vi "Sel Biometry Average Standard Deviation.vi"(8 "error in (no error)":errorcluster caption="错误输入（无错误）", 9 "condition":string, 11 "connection reference":T2) -> (0 "error out":errorcluster caption="错误输出", 2 "Biometry_Average_Standard_Deviation":T1[](array[typedef]))   [LabVIEW 2015, in "Database Processing.lvlib"]
doc: "该模板用于创建子VI。"
uses:
  Database Processing.lvlib
  <vilib>/addons/database/Connection.llb/Conn ObjectReference.ctl
  Support/Table/Biometry Average Standard Deviation.ctl
  <vilib>/addons/database/_DB Variant To Data/Database Variant To Data.xnode
  <vilib>/addons/database/NI_Database_API.lvlib
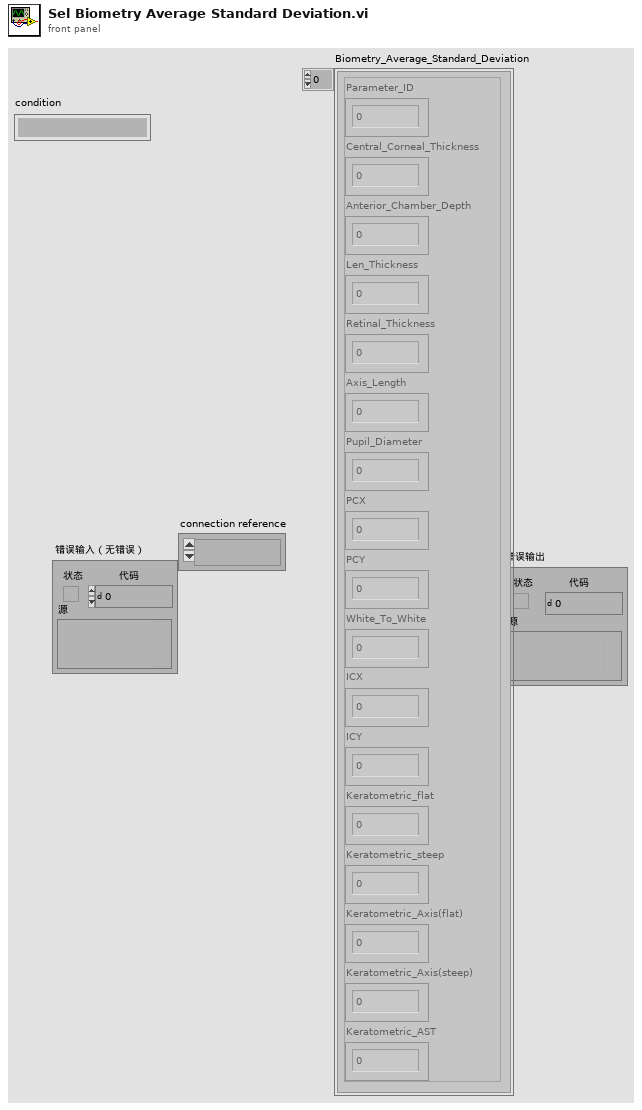
[diagram p1: front panel]
types:
  T1 = typedef "Database Processing.lvlib/Biometry Average Standard Deviation.ctl" = cluster{"Parameter_ID":i64, "Central_Corneal_Thickness":sgl, "Anterior_Chamber_Depth":sgl, "Len_Thickness":sgl, "Retinal_Thickness":sgl, "Axis_Length":sgl, "Pupil_Diameter":sgl, "PCX":sgl, "PCY":sgl, "White_To_White":sgl, "ICX":sgl, "ICY":sgl, "Keratometric_flat":sgl, "Keratometric_steep":sgl, "Keratometric_Axis(flat)":sgl, "Keratometric_Axis(steep)":sgl, "Keratometric_AST":sgl}
  T2 = typedef "NI_Database_API.lvlib/Conn ObjectReference.ctl" = refnum<k1>
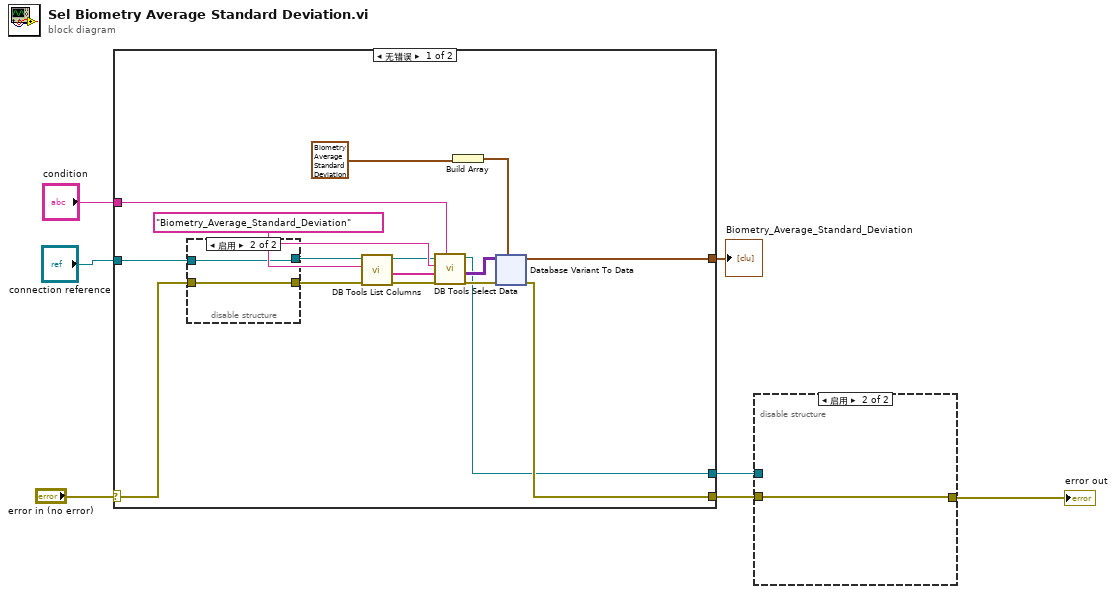
[diagram p0: block diagram]
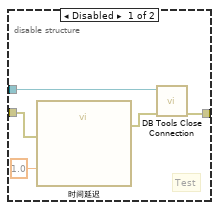
[diagram p2: hidden frame]
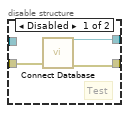
[diagram p3: hidden frame]
diagram:
  n1 = case shown="无错误" "error in (no error)" {
    selector: "error in (no error)" -> [w11 w567]
    tunnel: [w20 w567] -> w3
    tunnel: "connection reference" -> [w13 w566]
    tunnel: [w16 _] -> w1
    tunnel: "condition" -> [w15 _]
    tunnel: [w9 w566] -> w4
    frame No Error {
      w17 = "Biometry_Average_Standard_Deviation" ("table")
      n2 = disable-structure shown="启用" {
        disable-tunnel: [w26 w28] -> w14
        disable-tunnel: w13 -> [_ w28]
        disable-tunnel: w11 -> [w25 w27]
        disable-tunnel: [w24 w27] -> w12
        frame Disabled {
          # "Test"
          n3 = call "Connect Database.vi"("error in (no error)"=w25) -> ("error out"=w24:errorcluster, "connection reference"=w26:T2)  [unwired: 9 in]
        }
        frame Enabled {
        }
      }
      n4 = call <vilib>:"DB Tools List Columns.vi"("error in (no error)"=w12, "table"=w17, "connection reference"=w14) -> ("error out"=w19:errorcluster, "columns"=w18:string[], "connection reference out"=w10:T2)  [unwired: 1 in, 1 out]
      n5 = call <vilib>:"DB Tools Select Data.vi"("condition"=w15, "error in (no error)"=w19, "columns"=w18, "table"=w17, "connection reference"=w10) -> ("error out"=w23:errorcluster, "data"=w22:variant[][], "connection reference out"=w9:T2)  [unwired: 1 in]
      n6 = Build Array(T1 {"Parameter_ID"=0, "Central_Corneal_Thickness"=0.0, "Anterior_Chamber_Depth"=0.0, "Len_Thickness"=0.0, "Retinal_Thickness"=0.0, "Axis_Length"=0.0, "Pupil_Diameter"=0.0, "PCX"=0.0, "PCY"=0.0, "White_To_White"=0.0, "ICX"=0.0, "ICY"=0.0, "Keratometric_flat"=0.0, "Keratometric_steep"=0.0, "Keratometric_Axis(flat)"=0.0, "Keratometric_Axis(steep)"=0.0, "Keratometric_AST"=0.0} ("Biometry Average Standard Deviation")) -> (w21:T1[])
      n7 = xnode "Database Variant To Data"("database variant"=w22, "error in (no error)"=w23, "type"=w21) -> ("data"=w16:T1[], "error out"=w20:errorcluster)
    }
    frame Error {
    }
  }
  "Biometry_Average_Standard_Deviation" <- w1
  n8 = disable-structure shown="启用" {
    disable-tunnel: w3 -> [w570 w573]
    disable-tunnel: [w572 w573] -> w2
    disable-tunnel: w4 -> [w571 _]
    frame Disabled {
      # "Test"
      n9 = call "时间延迟"("error in (no error)"=w570, "Delay Time (s)"=1.0) -> ("error out"=w569:errorcluster)  [unwired: 9 in]
      n10 = call <vilib>:"DB Tools Close Connection.vi"("error in (no error)"=w569, "connection reference"=w571) -> ("error out"=w572:errorcluster)  [unwired: 5 in]
    }
    frame Enabled {
    }
  }
  "error out" <- w2
